vi "Paired_cosine_distances.vi"(8 "error in":errorcluster caption="entrée d'erreur", 10 "Y":string[][](array[string]), 11 "X":string[][](array[string])) -> (0 "error out":errorcluster caption="sortie d'erreur", 3 "Data":T1)   [LabVIEW 2020]
doc: "Computes the paired cosine distances between X and Y\n\nParameters :\n\n- X : array-like, shape (n_samples, n_features)\n\n- Y : array-like, shape (n_samples, n_features)\n\nReturns : \n\n- distances : ndarray, shape (n_samples, )"
uses:
  Paired_cosine_distances.lvclass
panel:
  out "Paired_cosine_distances.lvclass":refnum<class "Paired_cosine_distances.lvclass">
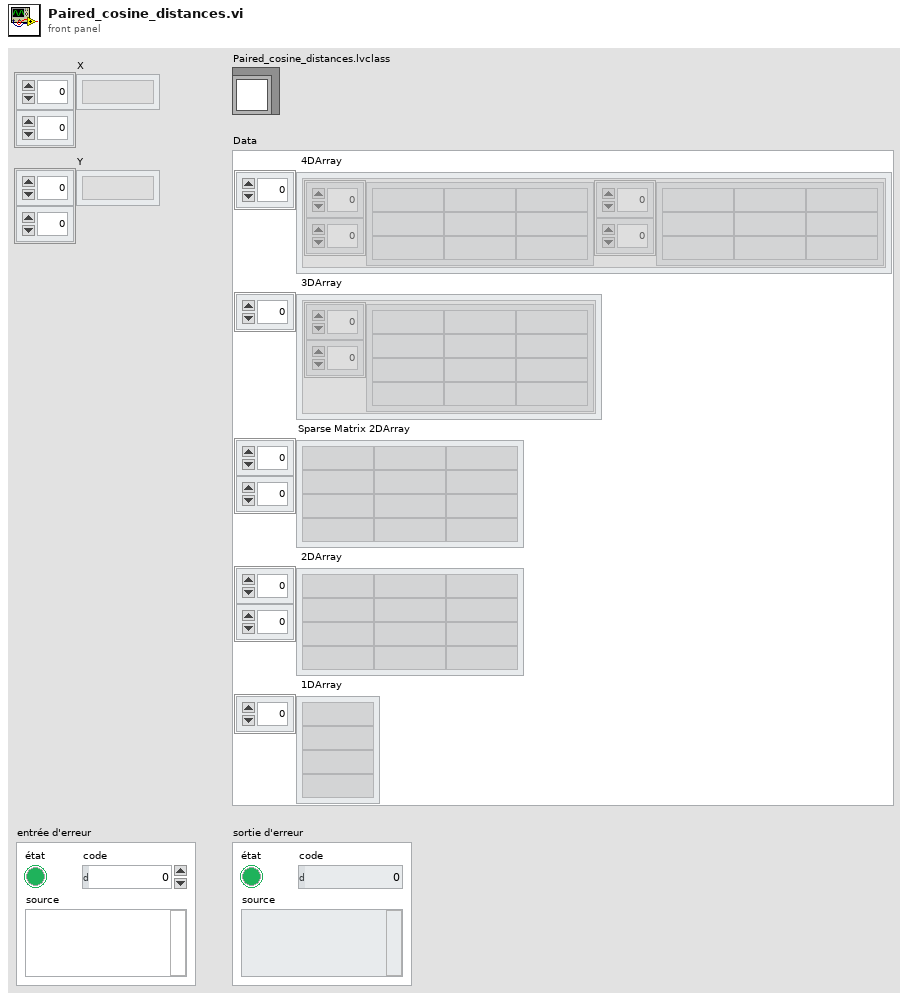
[diagram p1: front panel]
types:
  T1 = cluster{" 4DArray":cluster{"1":string[][], "2":string[][]}[], " 3DArray":cluster{"Tableau":string[][]}[], "Sparse Matrix 2DArray":string[][], " 2DArray":string[][], " 1DArray":string[]}
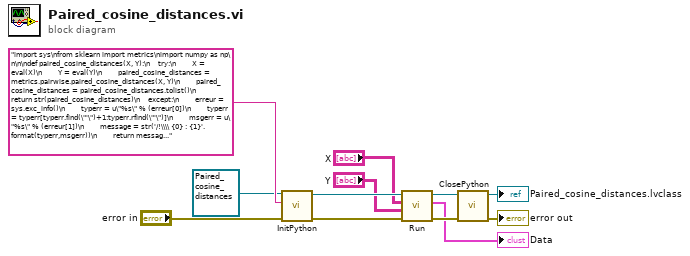
[diagram p0: block diagram]
diagram:
  n1 = call-dynamic "InitPython.vi"("error in (no error)"="error in", "Python Instruction"="import sys\nfrom sklearn import metrics\nimport numpy as np\n\n\ndef paired_cosine_distances(X, Y):\n    try:\n        X = eval(X)\n        Y = eval(Y)\n        paired_cosine_distances = metrics.pairwise.paired_cosine_distances(X, Y)\n        paired_cosine_distances = paired_cosine_distances.tolist()\n        return str(paired_cosine_distances)\n    except:\n        erreur = sys.exc_info()\n        typerr = u\"%s\" % (erreur[0])\n        typerr = typerr[typerr.find(\"'\")+1:typerr.rfind(\"'\")]\n        msgerr = u\"%s\" % (erreur[1])\n        message = str('/!\\\\ {0} : {1}'. format(typerr,msgerr))\n        return message", "Scikit-learn en entrée"=refnum<class "Paired_cosine_distances.lvclass"> refnum ("Paired_cosine_distances.lvclass")) -> ("error out"=w8:errorcluster, "Scikit-learn en sortie"=w9:refnum<class "Paired_cosine_distances.lvclass">)  [unwired: 7 in]
  n2 = call-dynamic "Run.vi"("error in (no error)"=w8, "Y"="Y", "X"="X", "Paired_cosine_distances.lvclass"=w9) -> ("error out"=w7:errorcluster, "Data"=→"Data":T1, "Paired_cosine_distances.lvclass"=w6:refnum<class "Paired_cosine_distances.lvclass">)  [unwired: 5 in]
  n3 = call-dynamic "ClosePython.vi"("error in (no error)"=w7, "Scikit-learn en entrée"=w6) -> ("error out"=→"error out":errorcluster, "Scikit-learn en sortie"=→"Paired_cosine_distances.lvclass":refnum<class "Paired_cosine_distances.lvclass">)  [unwired: 8 in]
